vi "MatLab-LV.vi"(10 "data in":string) -> (2 "data out":string)   [LabVIEW 2022 SP3]
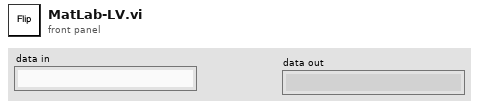
[diagram p1: front panel]
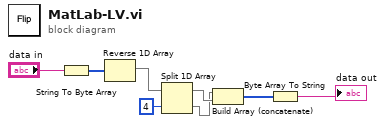
[diagram p0: block diagram]
diagram:
  n1 = String To Byte Array(string="data in") -> (unsigned byte array=w8:u8[])
  n2 = Reverse 1D Array(array=w8) -> (reversed array=w5:u8[])
  n3 = Split 1D Array(array=w5, index=4) -> (first subarray=w3:u8[], second subarray=w2:u8[])
  n4 = Build Array (concatenate)(w2, w3) -> (w1:u8[])
  n5 = Byte Array To String(unsigned byte array=w1) -> (string=→"data out":string)
